vi "Instrument Options.vi"(8 "error in (no error)":errorcluster, 11 "VISA resource name":refnum<visa-resource-name>) -> (0 "error out":errorcluster, 1 "Options List":string, 3 "VISA resource name out":refnum<visa-resource-name>)   [LabVIEW 2015, in "Rohde&Schwarz CMXP NR FR2 Measurement.lvlib"]
doc: "This VI returns the instrument version number and the list of options which the instrument is equipped with.\n\nRemote-control commands:\n*IDN?\n*OPT?"
uses:
  <instrlib>/Rohde&Schwarz CMXP NR FR2 Measurement/Rohde&Schwarz CMXP NR FR2 Measurement.lvlib
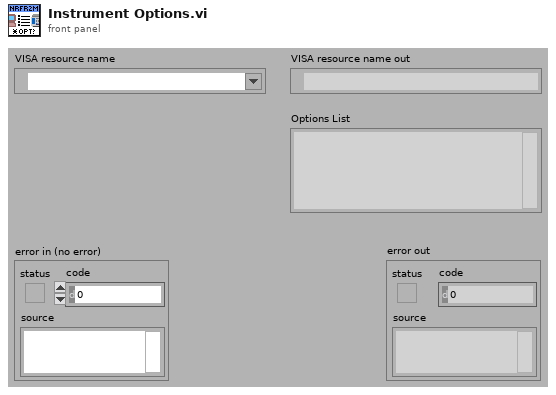
[diagram p1: front panel]
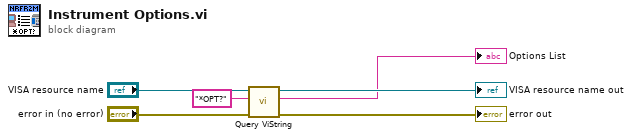
[diagram p0: block diagram]
diagram:
  n1 = call <instrlib>:"Query ViString.vi"("error in (no error)"="error in (no error)", "Query"="*OPT?", "VISA resource name"="VISA resource name") -> ("error out"=→"error out":errorcluster, "Response Value"=→"Options List":string, "VISA resource name out"=→"VISA resource name out":refnum<visa-resource-name>)  [unwired: 6 in]
